vi "Target Step Counter.vi"(11 "HS":bool) -> (3 "Number of Steps":i64)   [LabVIEW 2018, in "COBRA Iterative Learning Control Library.lvlib"]
uses:
  COBRA Iterative Learning Control Library.lvlib
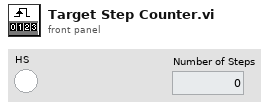
[diagram p1: front panel]
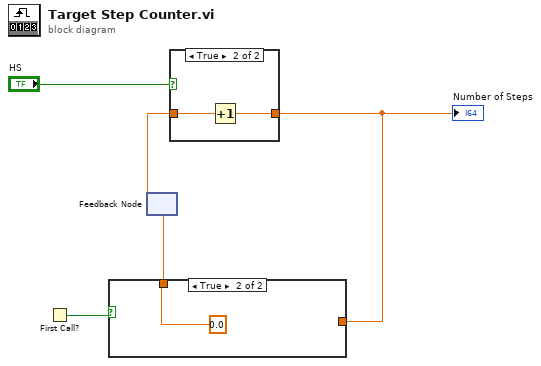
[diagram p0: block diagram]
diagram:
  n1 = First Call?() -> (First Call?: T/F=w3:bool)
  n2 = feedback #1() -> (w4:dbl)  [unwired: 1 in]
  n3 = case shown="True" "HS" {
    tunnel: [w6 w8] -> w1
    tunnel: w4 -> [w6 w7]
    frame False {
    }
    frame True {
      n4 = Increment(x=w7) -> (x+1=w8:dbl)
    }
  }
  "Number of Steps" <- w1
  n5 = case shown="True" w3 {
    tunnel: [w9 0.0] -> w2
    tunnel: w1 -> [w9 _]
    frame False {
    }
    frame True {
    }
  }
  n6 = feedback-in #1(w2) -> ()
